vi "Read channels.vi"(8 "error in (no error)":errorcluster, 11 "Wait On Boolean Step Config in":refnum<class "Wait On Boolean Step Config.lvclass">) -> (0 "error out":errorcluster, 2 "Channels":refnum<class "TBM channel.lvclass">[](array[class]), 3 "Wait On Boolean Step Config out":refnum<class "Wait On Boolean Step Config.lvclass">)   [LabVIEW 2015, in "Wait On Boolean Step Config.lvclass"]
uses:
  Wait On Boolean Step Config.lvclass
  <vilib>/NI/Tag Bus Module Framework/channel/TBM channel.lvclass
  Wait On Boolean Step Config.lvclass/Wait On Boolean Step Config.ctl
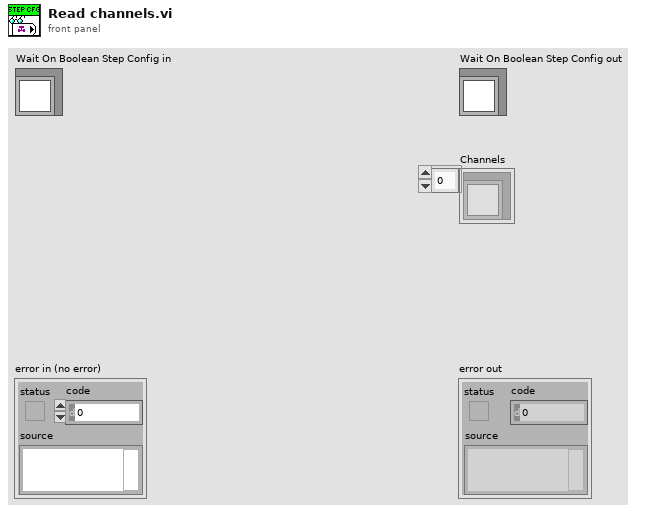
[diagram p1: front panel]
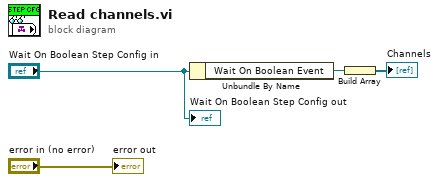
[diagram p0: block diagram]
diagram:
  n1 = Unbundle By Name("Wait On Boolean Step Config in") -> ("Wait On Boolean Event"=w4:refnum<class "TBM channel.lvclass">)
  n2 = Build Array(w4) -> (→"Channels":refnum<class "TBM channel.lvclass">[])
  "error out" <- "error in (no error)"
  "Wait On Boolean Step Config out" <- "Wait On Boolean Step Config in"
